vi "ZhiYuan ZDS Series for TCP Transfer Current Waveform(Support big timebase).vi"() -> ()   [LabVIEW 2015]
doc: "This example shows how to transfer the current waveform using Single mode on an oscilloscope, support read waveform in big timebase. Users can setup the acquired waveform using the instrument's front panel interface and then transfer that waveform to the computer using this example."
uses:
  ZhiYuan ZDS Series for TCP.lvlib
panel:
  in  "Maximum Waveform Point":i32(ring)=3 items=["14000"=1, "140000"=2, "1400000"=3, "14000000"=4, "56000000"=5]
  in  "Timeout (ms)":u32=5000
  out "Waveform Data":dbl[](graph)
  in  "Channel":u16(ring)=1 items=["Channel 1"=1, "Channel 2"=2, "Channel 3"=3, "Channel 4"=4]
  in  "VISA resource name":refnum<visa-resource-name>
  # "(c) 2012 National Instruments.  ALL RIGHTS RESERVED."
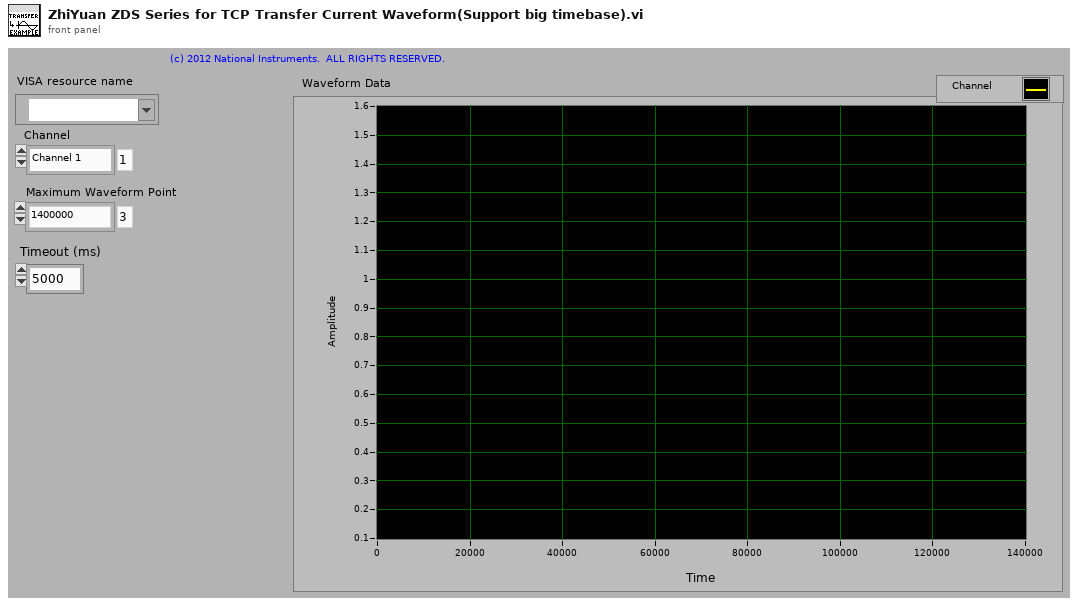
[diagram p1: front panel]
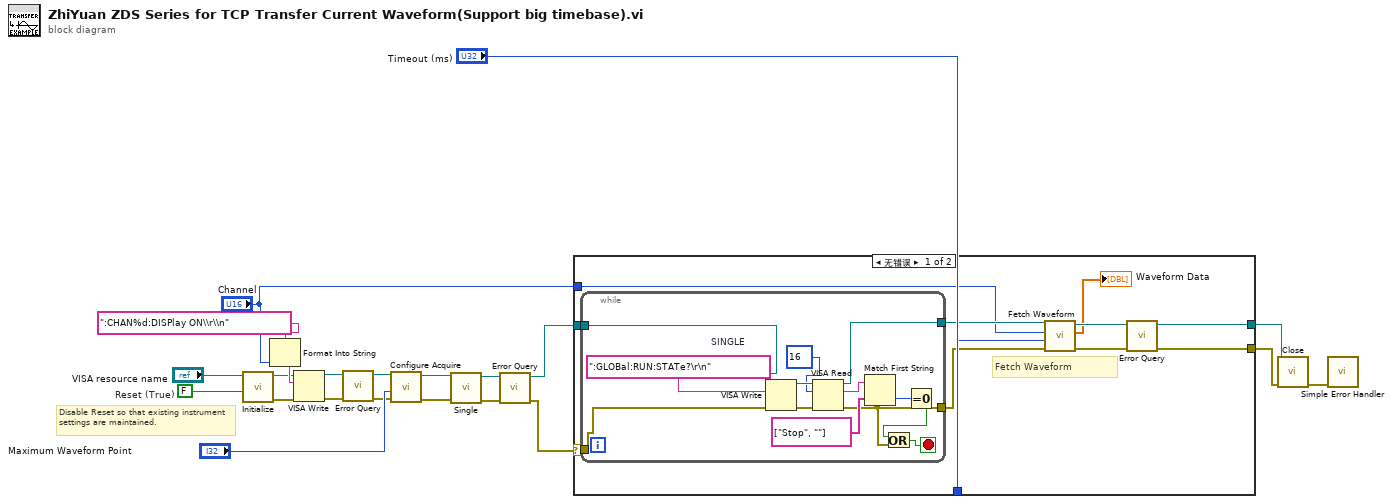
[diagram p0: block diagram]
diagram:
  w21 = FALSE  # Reset (True)
  # "Disable Reset so that existing instrument settings are maintained."
  n1 = call "Initialize.vi"("Reset (True)"=w21, "VISA resource name"="VISA resource name") -> ("error out"=w12:errorcluster, "VISA resource name out"=w13:refnum<visa-resource-name>)  [unwired: 8 in]
  n2 = Format Into String(format string=":CHAN%d:DISPlay ON\\r\\n", "Channel") -> (resulting string=w14:string)  [unwired: 2 in, 1 out]
  n3 = VISA Write(VISA resource name=w13, write buffer=w14, error in (no error)=w12) -> (VISA resource name out=w11:refnum<visa-resource-name>, error out=w15:errorcluster)  [unwired: 1 out]
  n4 = call "Error Query.vi"("error in (no error)"=w15, "VISA resource name"=w11) -> ("error out"=w9:errorcluster, "VISA resource name out"=w10:refnum<visa-resource-name>)  [unwired: 6 in, 2 out]
  n5 = call "Configure Acquire.vi"("error in (no error)"=w9, "Waveform Point Number (0: Auto)"="Maximum Waveform Point", "VISA resource name"=w10) -> ("error out"=w20:errorcluster, "VISA resource name out"=w19:refnum<visa-resource-name>)  [unwired: 7 in]
  n6 = call "Single.vi"("error in (no error)"=w20, "VISA resource name"=w19) -> ("error out"=w18:errorcluster, "VISA resource name out"=w17:refnum<visa-resource-name>)  [unwired: 8 in]
  n7 = call "Error Query.vi"("error in (no error)"=w18, "VISA resource name"=w17) -> ("error out"=w2:errorcluster, "VISA resource name out"=w7:refnum<visa-resource-name>)  [unwired: 6 in, 2 out]
  n8 = case shown="无错误" w2 {
    selector: w2 -> [w23 w48]
    tunnel: w7 -> [w29 w47]
    tunnel: "Timeout (ms)" -> [w28 _]
    tunnel: "Channel" -> [w27 _]
    tunnel: [w26 w48] -> w4
    tunnel: [w25 w47] -> w3
    frame No Error {
      # "Fetch Waveform"
      n9 = while {
        tunnel: w29 -> [w42]
        tunnel: [w41] -> w32
        tunnel: [w35] -> w33
        tunnel: w23 -> [w37]
        stop <- w34 stop-if-true
        w46 = ":GLOBal:RUN:STATe?\r\n"  # SINGLE
        n10 = VISA Write(VISA resource name=w42, write buffer=w46, error in (no error)=w37) -> (VISA resource name out=w44:refnum<visa-resource-name>, error out=w45:errorcluster)  [unwired: 1 out]
        n11 = VISA Read(VISA resource name=w44, byte count=16, error in (no error)=w45) -> (VISA resource name out=w41:refnum<visa-resource-name>, read buffer=w38:string, error out=w35:errorcluster)  [unwired: 1 out]
        n12 = Match First String(2:string[] ["Stop", ""], 3:w38) -> (0:w40:i32)  [unwired: 1 out]
        n13 = Equal To 0?(x=w40) -> (x = 0?=w36:bool)
        n14 = Or(x=w36, y=w35) -> (x .or. y?=w34:bool)
      }
      n15 = call "Fetch Waveform.vi"("error in (no error)"=w33, "Timeout (5000 ms)"=w28, "Channel (1: Channel 1)"=w27, "VISA resource name"=w32) -> ("error out"=w31:errorcluster, "Waveform Data"=→"Waveform Data":dbl[], "VISA resource name out"=w30:refnum<visa-resource-name>)  [unwired: 5 in]
      n16 = call "Error Query.vi"("error in (no error)"=w31, "VISA resource name"=w30) -> ("error out"=w26:errorcluster, "VISA resource name out"=w25:refnum<visa-resource-name>)  [unwired: 6 in, 2 out]
    }
    frame Error {
    }
  }
  n17 = call "Close.vi"("error in (no error)"=w4, "VISA resource name"=w3) -> ("error out"=w1:errorcluster)  [unwired: 9 in]
  n18 = call <vilib>:"Simple Error Handler.vi"("error in (no error)"=w1) -> ()  [unwired: 4 in, 5 out]
